vi "DAQ_6212_trig_v2.vi"(0 "Port Used?":bool[](array[boolean])=[TRUE, TRUE, FALSE, FALSE, FALSE, FALSE, FALSE, FALSE], 1 "Initial":bool[](array[boolean])=[FALSE, FALSE, FALSE, FALSE, FALSE, FALSE, FALSE, FALSE], 2 "TTL Duration":u16=10 format="%.0f ms", 3 "device name":tag="Dev1", 4 "error in":errorcluster) -> (5 "errorout":errorcluster)   [LabVIEW 2012]
panel:
  # "CCD trig with NI DAQ"
  # "AO0"
  # "AO1"
  # "1 ms TTL is still detectable (iDus)"
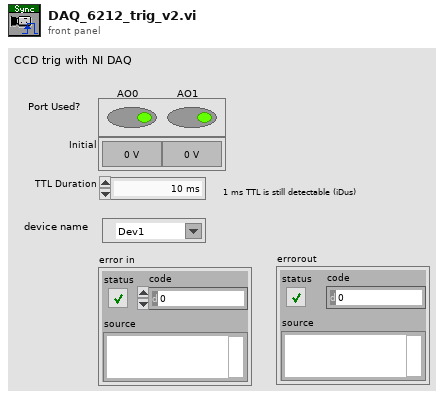
[diagram p1: front panel]
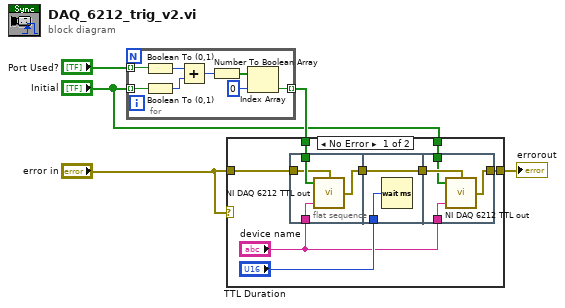
[diagram p0: block diagram]
diagram:
  n1 = for {
    tunnel: [w11] -> w5 mode=indexing
    tunnel: "Port Used?" -> [w7] mode=indexing
    tunnel: "Initial" -> [w6] mode=indexing
    n2 = Boolean To (0,1)(Boolean=w7) -> (0, 1=w10:i16)
    n3 = Boolean To (0,1)(Boolean=w6) -> (0, 1=w9:i16)
    n4 = Add(x=w10, y=w9) -> (x+y=w8:i16)
    n5 = Number To Boolean Array(number=w8) -> (Boolean array=w13:bool[])
    n6 = Index Array(array=w13, index=0) -> (element=w11:bool)
  }
  n7 = case shown="No Error" "error in" {
    tunnel: w5 -> [w21 _]
    tunnel: "error in" -> [w20 w32]
    tunnel: "Initial" -> [w15 _]
    tunnel: [w14 w32] -> w3
    frame No Error {
      n8 = flat-sequence {
        tunnel: w21 -> [w25]
        tunnel: "device name" -> [w24]
        tunnel: w20 -> [w23]
        tunnel: [w22] -> w19
        tunnel: w19 -> [w26]
        tunnel: "TTL Duration" -> [w27]
        tunnel: [w26] -> w17
        tunnel: w17 -> [w30]
        tunnel: "device name" -> [w31]
        tunnel: w15 -> [w29]
        tunnel: [w28] -> w14
        frame #0 {
          n9 = call "NI DAQ 6212 TTL out.vi"("error in"=w23, "device name"=w24, "data"=w25) -> ("errorout"=w22:errorcluster)  [unwired: 1 in]
        }
        frame #1 {
          n10 = Wait (ms)(milliseconds to wait=w27) -> ()  [unwired: 1 out]
        }
        frame #2 {
          n11 = call "NI DAQ 6212 TTL out.vi"("error in"=w30, "device name"=w31, "data"=w29) -> ("errorout"=w28:errorcluster)  [unwired: 1 in]
        }
      }
    }
    frame Error {
    }
  }
  "errorout" <- w3
